vi "GetAllDigitalInputs.vi"(4 "error in (no error)":errorcluster, 7 "axis in":cluster{"keyHandle":u32, "nodeId":u16}={"keyHandle"=0, "nodeId"=1}) -> (0 "error out":errorcluster, 2 "digital inputs":T1, 3 "axis out":cluster{"keyHandle":u32, "nodeId":u16}={"keyHandle"=0, "nodeId"=1})   [LabVIEW 2019, in "maxonEPOS.lvlib"]
doc: "<B>GetAllDigitalInputs</B> reads the state of all digital inputs from the device."
uses:
  Examples/maxonEPOS.lvlib
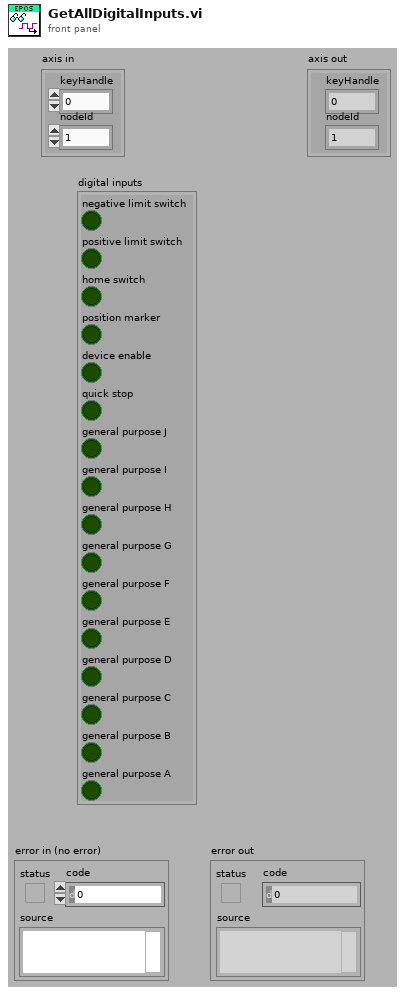
[diagram p1: front panel]
types:
  T1 = cluster{"negative limit switch":bool, "positive limit switch":bool, "home switch":bool, "position marker":bool, "device enable":bool, "quick stop":bool, "general purpose J":bool, "general purpose I":bool, "general purpose H":bool, "general purpose G":bool, "general purpose F":bool, "general purpose E":bool, "general purpose D":bool, "general purpose C":bool, "general purpose B":bool, "general purpose A":bool}
  T2 = cluster{"Boolean array[0]":bool, "Boolean array[1]":bool, "Boolean array[2]":bool, "Boolean array[3]":bool, "Boolean array[4]":bool, "Boolean array[5]":bool, "Boolean array[6]":bool, "Boolean array[7]":bool, "Boolean array[8]":bool, "Boolean array[9]":bool, "Boolean array[10]":bool, "Boolean array[11]":bool, "Boolean array[12]":bool, "Boolean array[13]":bool, "Boolean array[14]":bool, "Boolean array[15]":bool}
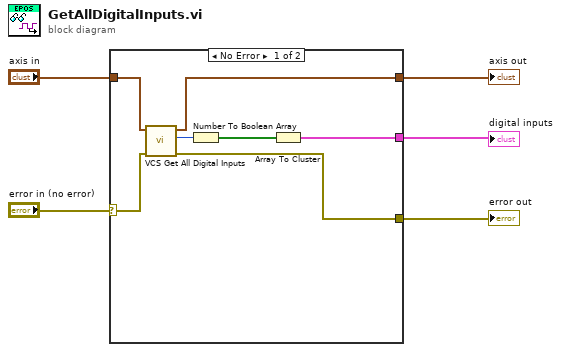
[diagram p0: block diagram]
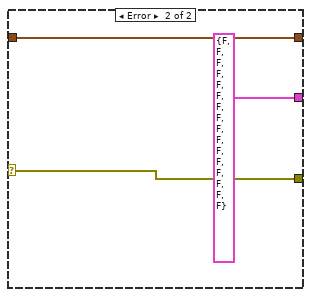
[diagram p2: hidden frame]
diagram:
  n1 = case shown="No Error" "error in (no error)" {
    selector: "error in (no error)" -> [w8 w15]
    tunnel: [w7 w15] -> w4
    tunnel: [w6 w14] -> w3
    tunnel: "axis in" -> [w12 w14]
    tunnel: [w9 T2 {"Boolean array[0]"=FALSE, "Boolean array[1]"=FALSE, "Boolean array[2]"=FALSE, "Boolean array[3]"=FALSE, "Boolean array[4]"=FALSE, "Boolean array[5]"=FALSE, "Boolean array[6]"=FALSE, "Boolean array[7]"=FALSE, "Boolean array[8]"=FALSE, "Boolean array[9]"=FALSE, "Boolean array[10]"=FALSE, "Boolean array[11]"=FALSE, "Boolean array[12]"=FALSE, "Boolean array[13]"=FALSE, "Boolean array[14]"=FALSE, "Boolean array[15]"=FALSE} ("Boolean array")] -> w1
    frame No Error {
      n2 = call "VCS Get All Digital Inputs.vi"("error in (no error)"=w8, "axis in"=w12) -> ("error out"=w7:errorcluster, "digital inputs"=w11:u16, "axis out"=w6:cluster{"keyHandle":u32, "nodeId":u16})  [unwired: 7 in]
      n3 = Number To Boolean Array(number=w11) -> (Boolean array=w10:bool[])
      n4 = Array To Cluster(array=w10) -> (cluster=w9:T2)
    }
    frame Error {
    }
  }
  "error out" <- w4
  "axis out" <- w3
  "digital inputs" <- w1
